vi "CANopenVM_57_single - 副本.vi"(0 "node-ID":u8=1 min=1 max=127 step=1, 1 "目标速度":i16=50) -> (2 "电机绝对位置":i32=443333152, 3 "速度反馈值":i32=300, 4 "转矩反馈值 0.1%":i16=40)   [LabVIEW 2020]
uses:
  <vilib>/Platform/TimedLoop/XDataNode/timing_clust.ctl
  <vilib>/Platform/TimedLoop/XDataNode/nitl_modes.ctl
  <vilib>/Platform/TimedLoop/XDataNode/wakeup.ctl
  <vilib>/CANopenLib/CANOPEN.llb/CANopen Interface Create.vi
  <vilib>/CANopenLib/CANOPEN.llb/CANopen SDO Create.vi
  <vilib>/CANopenLib/CANOPEN.llb/CANopen SDO Write [I16].vi
  <vilib>/CANopenLib/CANOPEN.llb/CANopen SDO Close.vi
  <vilib>/CANopenLib/CANOPEN.llb/CANopen SYNC Create.vi
  <vilib>/CANopenLib/CANOPEN.llb/CANopen RPDO Create.vi
  <vilib>/CANopenLib/CANOPEN.llb/CANopen TPDO Create.vi
  <vilib>/CANopenLib/CANOPEN.llb/CANopen TPDO Start.vi
  <vilib>/CANopenLib/CANOPEN.llb/CANopen SYNC Start.vi
  <vilib>/CANopenLib/CANOPEN.llb/CANopen RPDO Start.vi
  <vilib>/imath/engines/lvmath/Functions/Error Handling/MergeErrorsWrapper.vi
  <vilib>/imath/engines/lvmath2/RunTimeEngine/NodeEndStatement/NIMS_NodeEndStatement_Output.vi
  <instcachedir>/0/NIMS_NodeEndStatement_Output_53EC0D466D134D7ABD903AC30B43404B.lvgen/NIMS_NodeEndStatement_Output_53EC0D466D134D7ABD903AC30B43404B_010.vi
  <vilib>/imath/engines/lvmath2/RunTimeEngine/ErrorHandling/NIMS_Finalize Error.vi
  <vilib>/CANopenLib/CANOPEN.llb/CANopen Convert To Data [I16].vi
  <vilib>/CANopenLib/CANOPEN.llb/CANopen Fetch from Data [I16].vi
  <vilib>/CANopenLib/CANOPEN.llb/CANopen Fetch from Data [I32].vi
  <vilib>/CANopenLib/CANOPEN.llb/CANopen SYNC Close.vi
  <vilib>/CANopenLib/CANOPEN.llb/CANopen RPDO Close.vi
  <vilib>/CANopenLib/CANOPEN.llb/CANopen TPDO Close.vi
  <vilib>/CANopenLib/CANOPEN.llb/CANopen Interface Close.vi
  <vilib>/Platform/TimedLoop/XDataNode/XDataNode.xnode
  <vilib>/Platform/TimedLoop/XDataNode/XDNodeRunTimeDep.lvlib
panel:
  in  "node-ID  2":u8=1 min=1 max=127 step=1
  out "completion code 5":u32
  in  "buffer size (0) 4":u16
  in  "TPDO channel 2":u8(ring)=2 items=["PDO 1", "PDO 2", "PDO 3", "PDO 4"]
  in  "Set Target Vilocity 2":i16
  in  "stop 2":bool
  out "timestamp 2":timestamp=timestamp(3824613290.037175 s since 1904-01-01)
  out "电机绝对位置 2":i32=443333152
  out "速度反馈值 2":i32=300
  in  "目标速度  2":i16=50
  out "转矩反馈值 0.1% 2":i16=40
  in  "buffer size (0) 3":u16=10
  in  "TPDO channel read 2":u8(ring)=1 items=["PDO 1", "PDO 2", "PDO 3", "PDO 4"]
  in  "RPDO channel write 2":u8(ring)=1 items=["PDO 1", "PDO 2", "PDO 3", "PDO 4"]
  in  "period (ms) 2":i64=10
  out "completion code 4":u32
  out "completion code 3":u32
  in  "batch SDO name 2":string="NiMotion_VM"
  out "completion code":u32
  in  "buffer size (0) 2":u16
  in  "TPDO channel":u8(ring)=2 items=["PDO 1", "PDO 2", "PDO 3", "PDO 4"]
  in  "Set Target Vilocity":i16
  in  "stop":bool
  out "timestamp":timestamp=timestamp(3824613290.037175 s since 1904-01-01)
  in  "buffer size (0)":u16=10
  in  "TPDO channel read":u8(ring)=1 items=["PDO 1", "PDO 2", "PDO 3", "PDO 4"]
  in  "RPDO channel write":u8(ring)=1 items=["PDO 1", "PDO 2", "PDO 3", "PDO 4"]
  in  "period (ms)":i64=10
  out "completion code 2":u32
  out "completion code 1":u32
  in  "batch SDO name":string="NiMotion_VM"
  in  "baud rate":u32(ring) items=["1 Mbit/s"=0, "800 kbit/s"=1, "500 kbit/s"=2, "250 kbit/s"=3, "125 kbit/s"=4, "50 kbit/s"=6, "20 kbit/s"=7, "10 kbit/s"=8]
  in  "CANopen interface":u32(ring) items=["CANopen01", "CANopen02", "CANopen03", "CANopen04", "CANopen05", "CANopen06", "CANopen07", "CANopen08", "CANopen09", "CANopen10", "CANopen11", "CANopen12", "CANopen13", "CANopen14", "CANopen15", "CANopen16", "CANopen17", "CANopen18", "CANopen19", "CANopen20", "CANopen21", "CANopen22", "CANopen23", "CANopen24", "CANopen25", "CANopen26", "CANopen27", "CANopen28", "CANopen29", "CANopen30", "CANopen31", "CANopen32"]
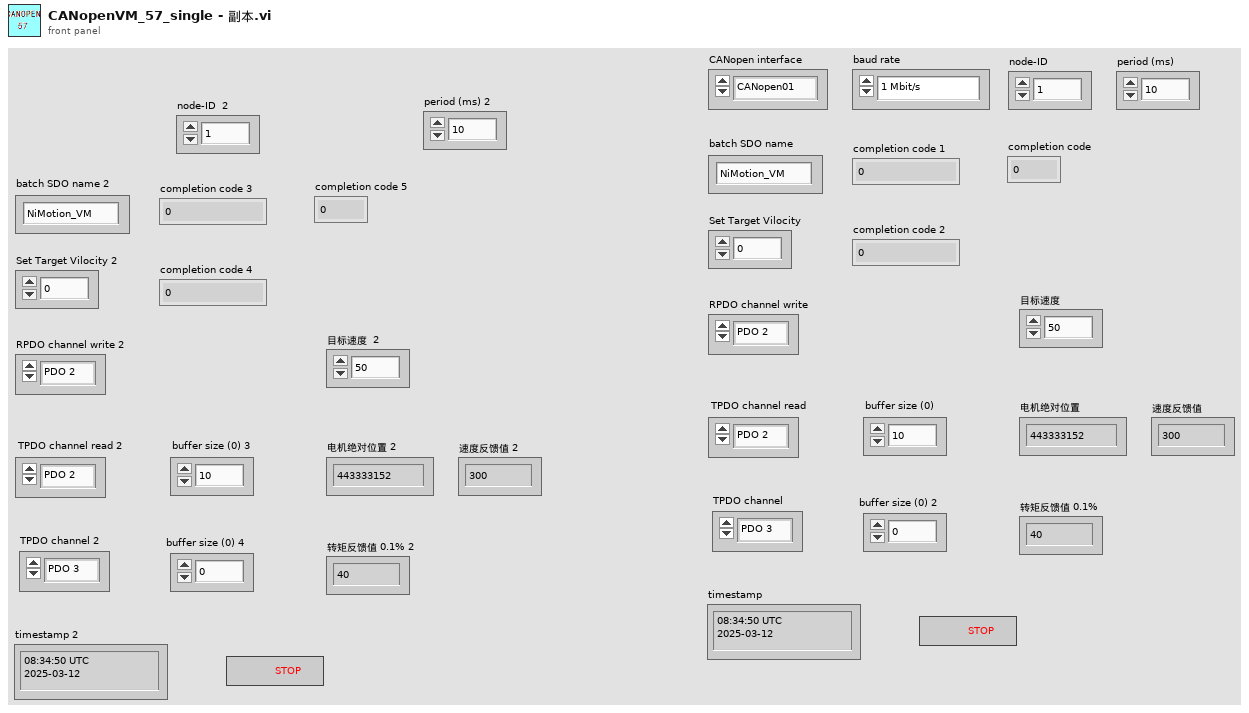
[diagram p1: front panel]
types:
  T1 = typedef "XDNodeRunTimeDep.lvlib/timing_clust.ctl" = cluster{"Expected End [f-1]":u64, "Actual End [f-1]":u64, "Finished Late? [f-1]":bool, "Expected End [i-1]":u64, "Actual End [i-1]":u64, "Finished Late? [i-1]":bool, "Expected Start [i]":u64, "Actual Start [i]":u64, "Expected Start [f]":u64, "Actual Start [f]":u64, "Source Name":string, "Structure Name":string, "Period":i64, "Deadline":i64, "Offset":i64, "Start":i64, "Priority":i32, "Timeout":i32, "Mode":T2, "Wakeup Reason":T3, "Error":errorcluster, "Source Type":string, "Secondary Source Type":string, "Global End Time":u64, "Global Start Time":u64, "Frame Duration":u64, "Iteration Duration":u64, "Assigned CPU":i32, "I/O Scan Engine Mode":u32}
  T2 = typedef "XDNodeRunTimeDep.lvlib/nitl_modes.ctl" = enum32{"No Change", "Process missed periods, maintain original phase", "Discard missed periods, maintain original phase", "Process missed periods, ignore original phase", "Discard missed periods, ignore original phase"}
  T3 = typedef "XDNodeRunTimeDep.lvlib/wakeup.ctl" = enum32{"Normal", "Aborted", "Asynchronous wakeup", "Timing source error", "Timed loop error", "Timeout"}
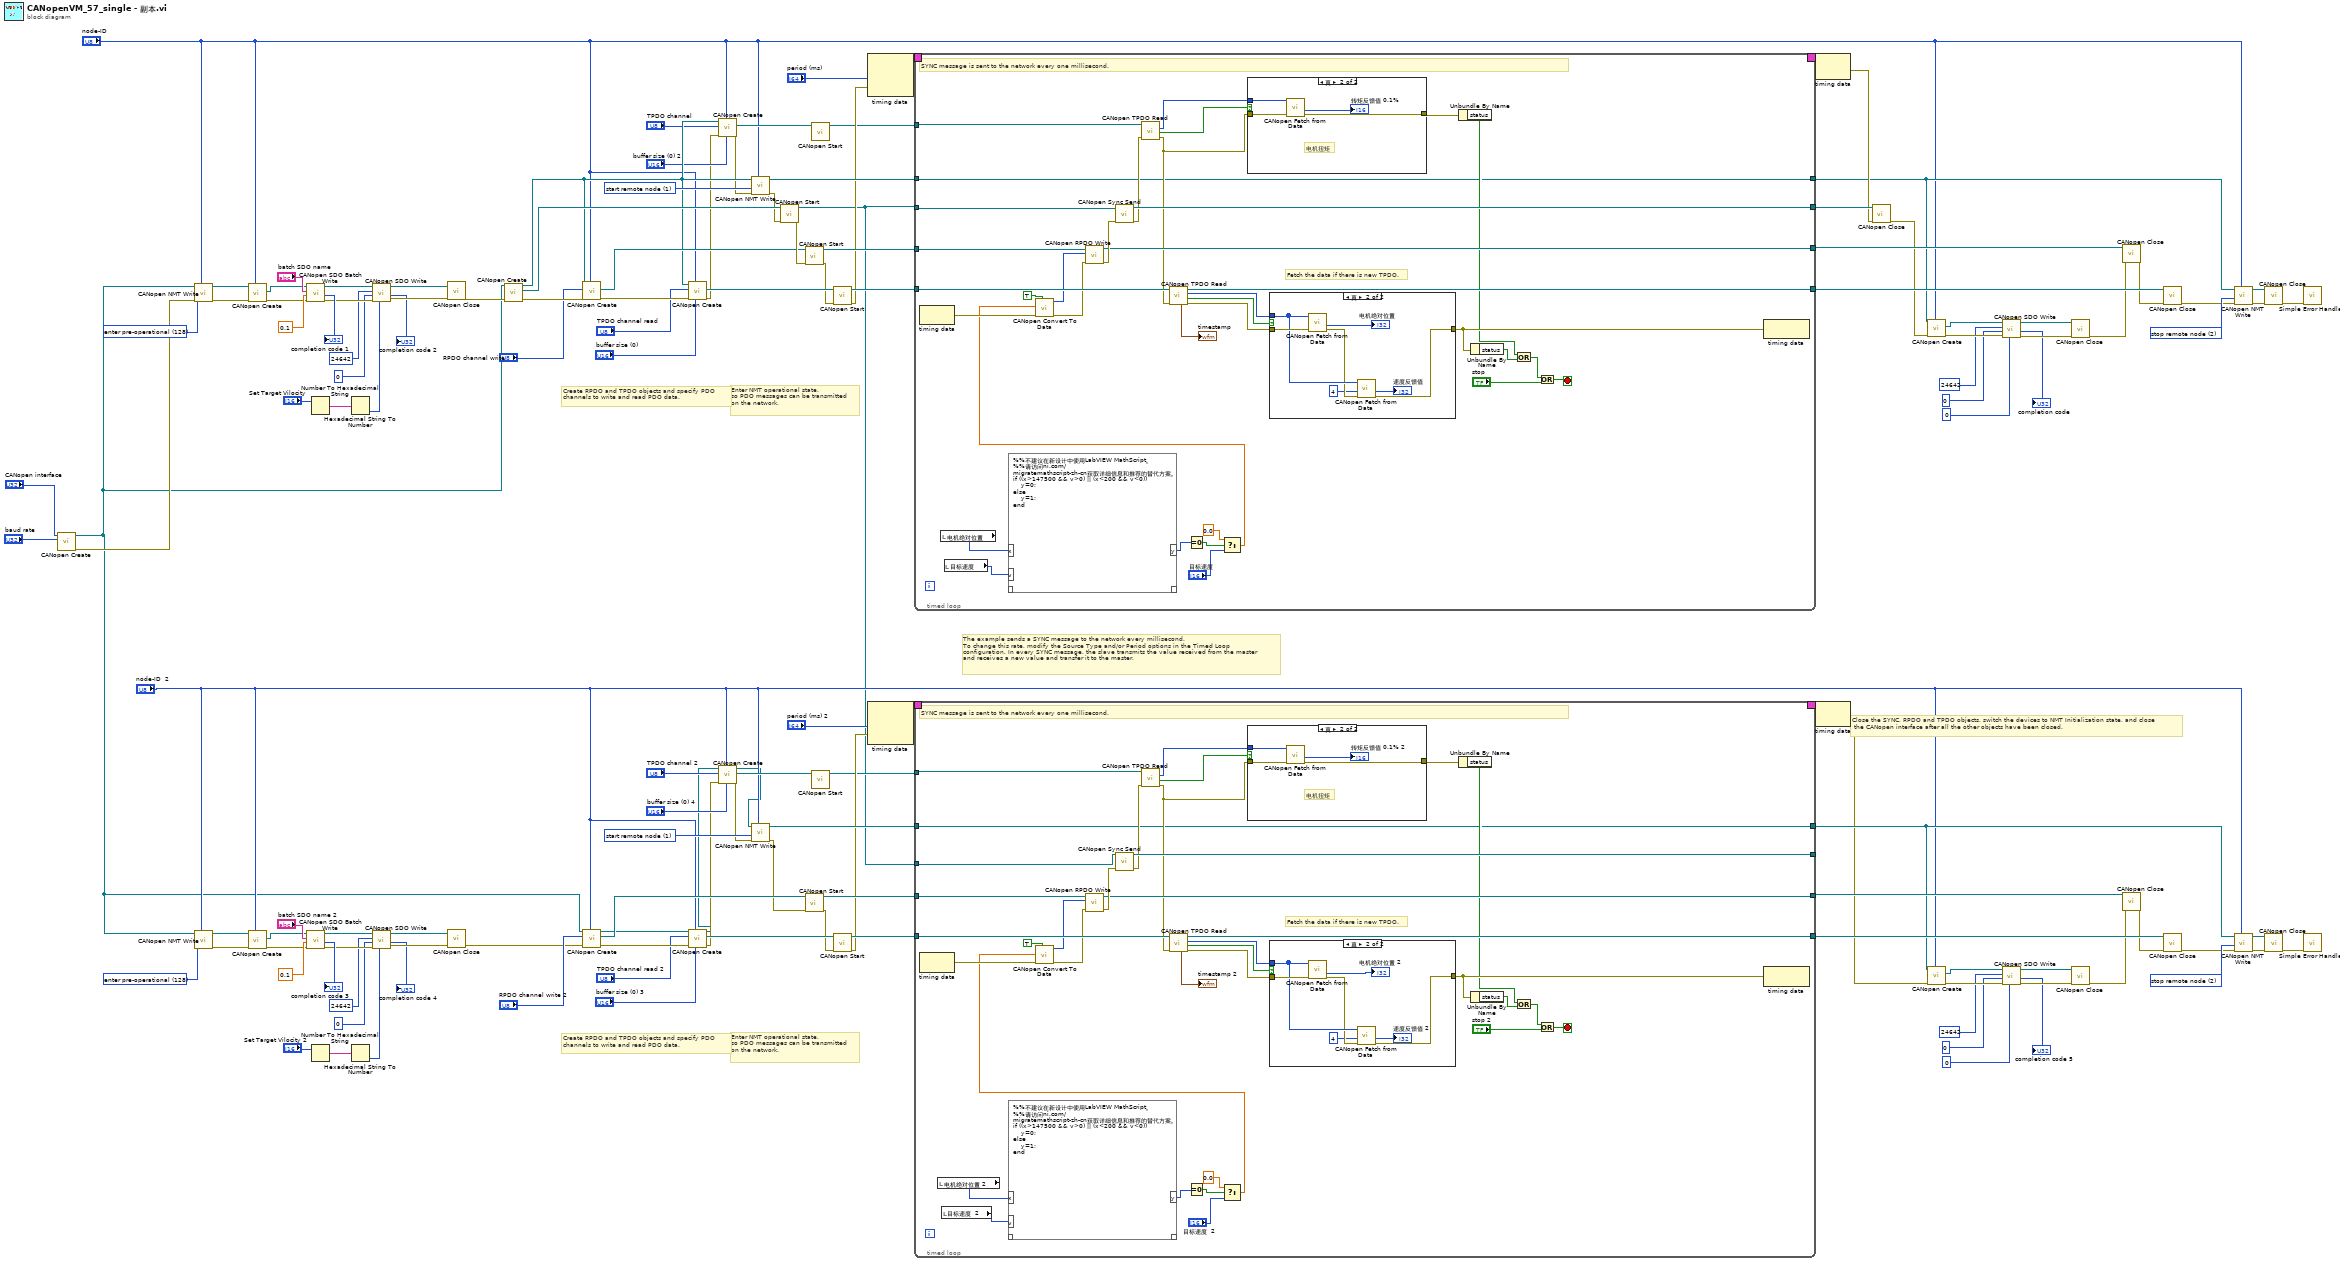
[diagram p0: block diagram]
diagram:
  w40 = u16 2 items=["start remote node"=1, "stop remote node"=2, "enter pre-operational"=128, "reset node"=129, "reset communication"=130] ("command")
  w48 = u16 1 items=["start remote node"=1, "stop remote node"=2, "enter pre-operational"=128, "reset node"=129, "reset communication"=130] ("command")
  w62 = u16 128 items=["start remote node"=1, "stop remote node"=2, "enter pre-operational"=128, "reset node"=129, "reset communication"=130] ("command")
  w102 = u16 2 items=["start remote node"=1, "stop remote node"=2, "enter pre-operational"=128, "reset node"=129, "reset communication"=130] ("command")
  w113 = u16 1 items=["start remote node"=1, "stop remote node"=2, "enter pre-operational"=128, "reset node"=129, "reset communication"=130] ("command")
  w129 = u16 128 items=["start remote node"=1, "stop remote node"=2, "enter pre-operational"=128, "reset node"=129, "reset communication"=130] ("command")
  # "SYNC message is sent to the network every one millisecond."
  # "Enter NMT operational state,\nso PDO messages can be transmitted\non the network."
  # "Create RPDO and TPDO objects and specify PDO \nchannels to write and read PDO data."
  # "SYNC message is sent to the network every one millisecond."
  # "Close the SYNC, RPDO and TPDO objects, switch the devices to NMT Initialization state, and close\n the CANopen interface after all the other objects have been closed."
  # "The example sends a SYNC message to the network every millisecond.\nTo change this rate, modify the Source Type and/or Period options in the Timed Loop\nconfiguration. In every SYNC message, the slave transmits the value received from the master\nand receives a new value and transfer it to the master."
  # "Enter NMT operational state,\nso PDO messages can be transmitted\non the network."
  # "Create RPDO and TPDO objects and specify PDO \nchannels to write and read PDO data."
  n1 = call-poly <vilib>:"CANopen Create.vi"("baud rate"="baud rate", "interface name"="CANopen interface") -> ("error out"=w130:errorcluster, "interface object out"=w7:refnum<k20>)  [unwired: 8 in]
  n2 = call <vilib>:"CANopen NMT Write.vi"("node-ID (0)"="node-ID", "error in (no error)"=w130, "command"=w129, "interface object in"=w7) -> ("error out"=w133:errorcluster, "interface object out"=w134:refnum<k20>)  [unwired: 6 in]
  n3 = call <vilib>:"CANopen NMT Write.vi"("node-ID (0)"="node-ID  2", "command"=w62, "interface object in"=w7) -> ("error out"=w63:errorcluster, "interface object out"=w64:refnum<k20>)  [unwired: 7 in]
  n4 = call-poly <vilib>:"CANopen Create.vi"("node-ID"="node-ID", "error in (no error)"=w133, "interface object in"=w134) -> ("error out"=w120:errorcluster, "SDO object out"=w126:refnum<k20>)  [unwired: 6 in, 1 out]
  n5 = call-poly <vilib>:"CANopen Create.vi"("node-ID"="node-ID  2", "error in (no error)"=w63, "interface object in"=w64) -> ("error out"=w53:errorcluster, "SDO object out"=w59:refnum<k20>)  [unwired: 6 in, 1 out]
  n6 = call <vilib>:"CANopen SDO Batch Write.vi"("error in (no error)"=w120, "timeout (1s)"=0.1 ("timeout (0s)"), "batch SDO name"="batch SDO name", "SDO object in"=w126) -> ("error out"=w121:errorcluster, "completion code"=→"completion code 1":u32, "SDO object out"=w124:refnum<k20>)  [unwired: 5 in]
  n7 = call <vilib>:"CANopen SDO Batch Write.vi"("error in (no error)"=w53, "timeout (1s)"=0.1 ("timeout (0s)"), "batch SDO name"="batch SDO name 2", "SDO object in"=w59) -> ("error out"=w54:errorcluster, "completion code"=→"completion code 3":u32, "SDO object out"=w57:refnum<k20>)  [unwired: 5 in]
  n8 = Number To Hexadecimal String(2:"Set Target Vilocity") -> (0:w90:string)  [unwired: 1 in]
  n9 = Number To Hexadecimal String(2:"Set Target Vilocity 2") -> (0:w30:string)  [unwired: 1 in]
  n10 = Hexadecimal String To Number(string=w90) -> (number=w88:u32)  [unwired: 2 in, 1 out]
  n11 = Hexadecimal String To Number(string=w30) -> (number=w28:u32)  [unwired: 2 in, 1 out]
  n12 = call-poly <vilib>:"CANopen SDO Write.vi"("I16 data"=w88, "error in (no error)"=w121, "object sub-index (0)"=u8 0, "object index"=u16 24642, "SDO object in"=w124) -> ("error out"=w122:errorcluster, "completion code"=→"completion code 2":u32, "SDO object out"=w123:refnum<k20>)  [unwired: 4 in]
  n13 = call-poly <vilib>:"CANopen SDO Write.vi"("I16 data"=w28, "error in (no error)"=w54, "object sub-index (0)"=u8 0, "object index"=u16 24642, "SDO object in"=w57) -> ("error out"=w55:errorcluster, "completion code"=→"completion code 4":u32, "SDO object out"=w56:refnum<k20>)  [unwired: 4 in]
  n14 = call-poly <vilib>:"CANopen Close.vi"("error in (no error)"=w122, "SDO object in"=w123) -> ("error out"=w105:errorcluster)  [unwired: 9 in]
  n15 = call-poly <vilib>:"CANopen Close.vi"("error in (no error)"=w55, "SDO object in"=w56) -> ("error out"=w8:errorcluster)  [unwired: 9 in]
  n16 = call-poly <vilib>:"CANopen Create.vi"("error in (no error)"=w105, "interface object in"=w7) -> ("error out"=w115:errorcluster, "SYNC object out"=w114:refnum<k20>, "interface object out"=w86:refnum<k20>)  [unwired: 7 in]
  n17 = call-poly <vilib>:"CANopen Create.vi"("node-ID"="node-ID", "error in (no error)"=w115, "PDO channel"="RPDO channel write", "interface object in"=w86) -> ("error out"=w109:errorcluster, "RPDO object out"=w108:refnum<k20>)  [unwired: 5 in, 1 out]
  n18 = call-poly <vilib>:"CANopen Create.vi"("node-ID"="node-ID  2", "error in (no error)"=w8, "PDO channel"="RPDO channel write 2", "interface object in"=w7) -> ("error out"=w46:errorcluster, "RPDO object out"=w45:refnum<k20>, "interface object out"=w6:refnum<k20>)  [unwired: 5 in]
  n19 = call-poly <vilib>:"CANopen Create.vi"("buffer size (0)"="buffer size (0)", "node-ID"="node-ID", "error in (no error)"=w109, "PDO channel"="TPDO channel read", "interface object in"=w86) -> ("error out"=w81:errorcluster, "TPDO object out"=w117:refnum<k20>)  [unwired: 4 in, 1 out]
  n20 = call-poly <vilib>:"CANopen Create.vi"("buffer size (0)"="buffer size (0) 3", "node-ID"="node-ID  2", "error in (no error)"=w46, "PDO channel"="TPDO channel read 2", "interface object in"=w6) -> ("error out"=w22:errorcluster, "TPDO object out"=w50:refnum<k20>, "interface object out"=w5:refnum<k20>)  [unwired: 4 in]
  n21 = call-poly <vilib>:"CANopen Create.vi"("buffer size (0)"="buffer size (0) 2", "node-ID"="node-ID", "error in (no error)"=w81, "PDO channel"="TPDO channel", "interface object in"=w86) -> ("error out"=w80:errorcluster, "TPDO object out"=w83:refnum<k20>)  [unwired: 4 in, 1 out]
  n22 = call-poly <vilib>:"CANopen Create.vi"("buffer size (0)"="buffer size (0) 4", "node-ID"="node-ID  2", "error in (no error)"=w22, "PDO channel"="TPDO channel 2", "interface object in"=w5) -> ("error out"=w21:errorcluster, "TPDO object out"=w24:refnum<k20>, "interface object out"=w4:refnum<k20>)  [unwired: 4 in]
  n23 = call <vilib>:"CANopen NMT Write.vi"("node-ID (0)"="node-ID", "error in (no error)"=w80, "command"=w113, "interface object in"=w86) -> ("error out"=w112:errorcluster, "interface object out"=w94:refnum<k20>)  [unwired: 6 in]
  n24 = call <vilib>:"CANopen NMT Write.vi"("node-ID (0)"="node-ID  2", "error in (no error)"=w21, "command"=w48, "interface object in"=w4) -> ("error out"=w3:errorcluster, "interface object out"=w34:refnum<k20>)  [unwired: 6 in]
  n25 = call-poly <vilib>:"CANopen Start.vi"("error in (no error)"=w112, "SYNC object in"=w114) -> ("error out"=w111:errorcluster, "SYNC object out"=w2:refnum<k20>)  [unwired: 8 in]
  n26 = call-poly <vilib>:"CANopen Start.vi"("error in (no error)"=w111, "RPDO object in"=w108) -> ("error out"=w110:errorcluster, "RPDO object out"=w93:refnum<k20>)  [unwired: 8 in]
  n27 = call-poly <vilib>:"CANopen Start.vi"("error in (no error)"=w3, "RPDO object in"=w45) -> ("error out"=w47:errorcluster, "RPDO object out"=w33:refnum<k20>)  [unwired: 8 in]
  n28 = call-poly <vilib>:"CANopen Start.vi"("TPDO object in"=w83) -> ("TPDO object out"=w82:refnum<k20>)  [unwired: 9 in, 1 out]
  n29 = call-poly <vilib>:"CANopen Start.vi"("TPDO object in"=w24) -> ("TPDO object out"=w23:refnum<k20>)  [unwired: 9 in, 1 out]
  n30 = call-poly <vilib>:"CANopen Start.vi"("error in (no error)"=w110, "TPDO object in"=w117) -> ("error out"=w91:errorcluster, "TPDO object out"=w92:refnum<k20>)  [unwired: 8 in]
  n31 = call-poly <vilib>:"CANopen Start.vi"("error in (no error)"=w47, "TPDO object in"=w50) -> ("error out"=w31:errorcluster, "TPDO object out"=w32:refnum<k20>)  [unwired: 8 in]
  n32 = node-c288("period (ms)", w91) -> (w136:T1)  [unwired: 1 in]
  n33 = node-c288("period (ms) 2", w31) -> (w66:T1)  [unwired: 1 in]
  n34 = timed-loop {
    timing: w136 -> [_]
    timing-out: [_] -> w135
    tunnel: w2 -> [w171]
    tunnel: [w161] -> w98
    tunnel: [w144] -> w78
    tunnel: w94 -> [w144]
    tunnel: w93 -> [w165]
    tunnel: w92 -> [w166]
    tunnel: [w163] -> w101
    tunnel: [w162] -> w79
    tunnel: w82 -> [w154]
    stop <- w170 stop-if-true
    # "Fetch the data if there is new TPDO."
    n35 = node-c288() -> (w156:errorcluster)  [unwired: 1 in]
    n36 = local read "电机绝对位置"() -> (w143:i32)
    n37 = local read "目标速度"() -> (w137:i16)
    n38 = mathscript code="%%不建议在新设计中使用LabVIEW MathScript。\n%%请访问ni.com/migratemathscript-zh-cn获取详细信息和推荐的替代方案。\nif ((x>147500 && v>0) || (x<200 && v<0))\n    y=0;\nelse\n    y=1;\nend"("x"=w143, "v"=w137) -> ("y"=w142:i32)  [unwired: 1 in, 1 out]
    n39 = Equal To 0?(x=w142) -> (x = 0?=w141:bool)
    n40 = Select(t=0.0, s=w141, f="目标速度") -> (s? t:f=w138:dbl)
    n41 = call-poly <vilib>:"CANopen Convert To Data.vi"("trim"=TRUE, "error in (no error)"=w156, "signed 16-bit integer"=w138) -> ("error out"=w145:errorcluster, "CANopen data out"=w155:u8[])  [unwired: 7 in]
    n42 = call <vilib>:"CANopen RPDO Write.vi"("error in (no error)"=w145, "data"=w155, "RPDO object in"=w165) -> ("error out"=w164:errorcluster, "RPDO object out"=w162:refnum<k20>)  [unwired: 7 in]
    n43 = call <vilib>:"CANopen Sync Send.vi"("error in (no error)"=w164, "SYNC object in"=w171) -> ("error out"=w153:errorcluster, "SYNC object out"=w161:refnum<k20>)  [unwired: 8 in]
    n44 = call <vilib>:"CANopen TPDO Read.vi"("error in (no error)"=w153, "TPDO object in"=w154) -> ("error out"=w150:errorcluster, "new data?"=w151:bool, "data"=w152:u8[])  [unwired: 5 in, 2 out]
    n45 = call <vilib>:"CANopen TPDO Read.vi"("error in (no error)"=w150, "TPDO object in"=w166) -> ("error out"=w167:errorcluster, "new data?"=w160:bool, "data"=w158:u8[], "TPDO object out"=w163:refnum<k20>, "timestamp"=→"timestamp":timestamp)  [unwired: 5 in]
    n46 = case shown="真" w151 {
      tunnel: w150 -> [w233 w237]
      tunnel: w152 -> [_ w236]
      tunnel: [w233 w235] -> w149
      frame False {
      }
      frame True {
        # "电机扭矩"
        n47 = call-poly <vilib>:"CANopen Fetch from Data.vi"("error in (no error)"=w237, "CANopen data in"=w236) -> ("error out"=w235:errorcluster, "signed 16-bit integer"=→"转矩反馈值 0.1%":i16)  [unwired: 7 in, 1 out]
      }
    }
    n48 = case shown="真" w160 {
      tunnel: w167 -> [w243 w250]
      tunnel: w158 -> [_ w249]
      tunnel: [w243 w247] -> w159
      frame False {
      }
      frame True {
        n49 = call-poly <vilib>:"CANopen Fetch from Data.vi"("error in (no error)"=w250, "CANopen data in"=w249) -> ("error out"=w248:errorcluster, "signed 32-bit integer"=→"电机绝对位置":i32)  [unwired: 7 in, 1 out]
        n50 = call-poly <vilib>:"CANopen Fetch from Data.vi"("error in (no error)"=w248, "offset (0)"=u32 4, "CANopen data in"=w249) -> ("error out"=w247:errorcluster, "signed 32-bit integer"=→"速度反馈值":i32)  [unwired: 6 in, 1 out]
      }
    }
    n51 = Unbundle By Name(w149) -> ("status"=w147:bool)
    n52 = Unbundle By Name(w159) -> ("status"=w148:bool)
    n53 = Or(x=w147, y=w148) -> (x .or. y?=w146:bool)
    n54 = Or(x=w146, y="stop") -> (x .or. y?=w170:bool)
    n55 = node-c288(w159) -> ()  [unwired: 1 out]
  }
  n56 = timed-loop {
    timing: w66 -> [_]
    timing-out: [_] -> w65
    tunnel: [w276] -> _
    tunnel: [w259] -> w19
    tunnel: w34 -> [w259]
    tunnel: w33 -> [w280]
    tunnel: w32 -> [w281]
    tunnel: [w278] -> w39
    tunnel: [w277] -> w20
    tunnel: w23 -> [w269]
    tunnel: w2 -> [w251]
    stop <- w285 stop-if-true
    # "Fetch the data if there is new TPDO."
    n57 = node-c288() -> (w271:errorcluster)  [unwired: 1 in]
    n58 = local read "电机绝对位置 2"() -> (w258:i32)
    n59 = local read "目标速度  2"() -> (w252:i16)
    n60 = mathscript code="%%不建议在新设计中使用LabVIEW MathScript。\n%%请访问ni.com/migratemathscript-zh-cn获取详细信息和推荐的替代方案。\nif ((x>147500 && v>0) || (x<200 && v<0))\n    y=0;\nelse\n    y=1;\nend"("x"=w258, "v"=w252) -> ("y"=w257:i32)  [unwired: 1 in, 1 out]
    n61 = Equal To 0?(x=w257) -> (x = 0?=w256:bool)
    n62 = Select(t=0.0, s=w256, f="目标速度  2") -> (s? t:f=w253:dbl)
    n63 = call-poly <vilib>:"CANopen Convert To Data.vi"("trim"=TRUE, "error in (no error)"=w271, "signed 16-bit integer"=w253) -> ("error out"=w260:errorcluster, "CANopen data out"=w270:u8[])  [unwired: 7 in]
    n64 = call <vilib>:"CANopen RPDO Write.vi"("error in (no error)"=w260, "data"=w270, "RPDO object in"=w280) -> ("error out"=w279:errorcluster, "RPDO object out"=w277:refnum<k20>)  [unwired: 7 in]
    n65 = call <vilib>:"CANopen Sync Send.vi"("error in (no error)"=w279, "SYNC object in"=w251) -> ("error out"=w268:errorcluster, "SYNC object out"=w276:refnum<k20>)  [unwired: 8 in]
    n66 = call <vilib>:"CANopen TPDO Read.vi"("error in (no error)"=w268, "TPDO object in"=w269) -> ("error out"=w265:errorcluster, "new data?"=w266:bool, "data"=w267:u8[])  [unwired: 5 in, 2 out]
    n67 = call <vilib>:"CANopen TPDO Read.vi"("error in (no error)"=w265, "TPDO object in"=w281) -> ("error out"=w282:errorcluster, "new data?"=w275:bool, "data"=w273:u8[], "TPDO object out"=w278:refnum<k20>, "timestamp"=→"timestamp 2":timestamp)  [unwired: 5 in]
    n68 = case shown="真" w266 {
      tunnel: w265 -> [w347 w351]
      tunnel: w267 -> [_ w350]
      tunnel: [w347 w349] -> w264
      frame False {
      }
      frame True {
        # "电机扭矩"
        n69 = call-poly <vilib>:"CANopen Fetch from Data.vi"("error in (no error)"=w351, "CANopen data in"=w350) -> ("error out"=w349:errorcluster, "signed 16-bit integer"=→"转矩反馈值 0.1% 2":i16)  [unwired: 7 in, 1 out]
      }
    }
    n70 = case shown="真" w275 {
      tunnel: w282 -> [w357 w364]
      tunnel: w273 -> [_ w363]
      tunnel: [w357 w361] -> w274
      frame False {
      }
      frame True {
        n71 = call-poly <vilib>:"CANopen Fetch from Data.vi"("error in (no error)"=w364, "CANopen data in"=w363) -> ("error out"=w362:errorcluster, "signed 32-bit integer"=→"电机绝对位置 2":i32)  [unwired: 7 in, 1 out]
        n72 = call-poly <vilib>:"CANopen Fetch from Data.vi"("error in (no error)"=w362, "offset (0)"=u32 4, "CANopen data in"=w363) -> ("error out"=w361:errorcluster, "signed 32-bit integer"=→"速度反馈值 2":i32)  [unwired: 6 in, 1 out]
      }
    }
    n73 = Unbundle By Name(w264) -> ("status"=w262:bool)
    n74 = Unbundle By Name(w274) -> ("status"=w263:bool)
    n75 = Or(x=w262, y=w263) -> (x .or. y?=w261:bool)
    n76 = Or(x=w261, y="stop 2") -> (x .or. y?=w285:bool)
    n77 = node-c288(w274) -> ()  [unwired: 1 out]
  }
  n78 = node-c288(w135) -> (w96:errorcluster)
  n79 = node-c288(w65) -> (w1:errorcluster)
  n80 = call-poly <vilib>:"CANopen Close.vi"("error in (no error)"=w96, "SYNC object in"=w98) -> ("error out"=w75:errorcluster)  [unwired: 9 in]
  n81 = call-poly <vilib>:"CANopen Create.vi"("node-ID"="node-ID", "error in (no error)"=w75, "interface object in"=w78) -> ("error out"=w74:errorcluster, "SDO object out"=w77:refnum<k20>)  [unwired: 6 in, 1 out]
  n82 = call-poly <vilib>:"CANopen Create.vi"("node-ID"="node-ID  2", "error in (no error)"=w1, "interface object in"=w19) -> ("error out"=w16:errorcluster, "SDO object out"=w18:refnum<k20>)  [unwired: 6 in, 1 out]
  n83 = call-poly <vilib>:"CANopen SDO Write.vi"("I16 data"=i16 0, "error in (no error)"=w74, "object sub-index (0)"=u8 0 ("sub-index"), "object index"=u16 24642, "SDO object in"=w77) -> ("error out"=w73:errorcluster, "completion code"=→"completion code":u32, "SDO object out"=w76:refnum<k20>)  [unwired: 4 in]
  n84 = call-poly <vilib>:"CANopen SDO Write.vi"("I16 data"=i16 0, "error in (no error)"=w16, "object sub-index (0)"=u8 0 ("sub-index"), "object index"=u16 24642, "SDO object in"=w18) -> ("error out"=w15:errorcluster, "completion code"=→"completion code 5":u32, "SDO object out"=w17:refnum<k20>)  [unwired: 4 in]
  n85 = call-poly <vilib>:"CANopen Close.vi"("error in (no error)"=w73, "SDO object in"=w76) -> ("error out"=w72:errorcluster)  [unwired: 9 in]
  n86 = call-poly <vilib>:"CANopen Close.vi"("error in (no error)"=w15, "SDO object in"=w17) -> ("error out"=w14:errorcluster)  [unwired: 9 in]
  n87 = call-poly <vilib>:"CANopen Close.vi"("error in (no error)"=w72, "RPDO object in"=w79) -> ("error out"=w100:errorcluster)  [unwired: 9 in]
  n88 = call-poly <vilib>:"CANopen Close.vi"("error in (no error)"=w14, "RPDO object in"=w20) -> ("error out"=w38:errorcluster)  [unwired: 9 in]
  n89 = call-poly <vilib>:"CANopen Close.vi"("error in (no error)"=w100, "TPDO object in"=w101) -> ("error out"=w99:errorcluster)  [unwired: 9 in]
  n90 = call-poly <vilib>:"CANopen Close.vi"("error in (no error)"=w38, "TPDO object in"=w39) -> ("error out"=w37:errorcluster)  [unwired: 9 in]
  n91 = call <vilib>:"CANopen NMT Write.vi"("node-ID (0)"="node-ID", "error in (no error)"=w99, "command"=w102, "interface object in"=w78) -> ("error out"=w104:errorcluster, "interface object out"=w103:refnum<k20>)  [unwired: 6 in]
  n92 = call <vilib>:"CANopen NMT Write.vi"("node-ID (0)"="node-ID  2", "error in (no error)"=w37, "command"=w40, "interface object in"=w19) -> ("error out"=w42:errorcluster, "interface object out"=w41:refnum<k20>)  [unwired: 6 in]
  n93 = call-poly <vilib>:"CANopen Close.vi"("error in (no error)"=w104, "interface object in"=w103) -> ("error out"=w97:errorcluster)  [unwired: 9 in]
  n94 = call-poly <vilib>:"CANopen Close.vi"("error in (no error)"=w42, "interface object in"=w41) -> ("error out"=w36:errorcluster)  [unwired: 9 in]
  n95 = call <vilib>:"Simple Error Handler.vi"("error in (no error)"=w97) -> ()  [unwired: 4 in, 5 out]
  n96 = call <vilib>:"Simple Error Handler.vi"("error in (no error)"=w36) -> ()  [unwired: 4 in, 5 out]
